vi "getStatus.vi"(8 "error in (no error)":errorcluster, 11 "SpinCore in":refnum<class "SpinCore.lvclass">) -> (0 "error out":errorcluster, 2 "status array":bool[](array[boolean]), 3 "SpinCore out":refnum<class "SpinCore.lvclass">)   [LabVIEW 2009, in "Hardware.lvlib" / "Channels.lvlib" / "SpinCore.lvclass"]
uses:
  SpinCore.lvclass
  SpinCore.lvclass/SpinCore.ctl
panel:
  # "pb_read_status(void) returns a 32 bit int:\nbit0 :stopped\nbit1: Reset\nbit2:Running\nbit3: Waiting\nBit4: Scanning (not this board)\nBit5-31 are reserved for future use.\n\nSee SpinAPI reference for details"
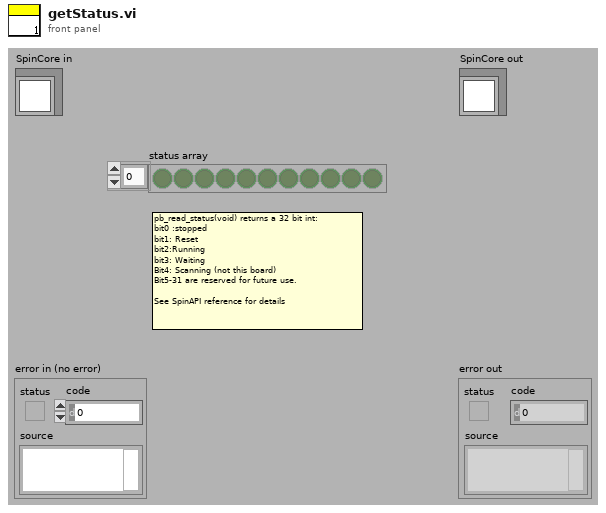
[diagram p1: front panel]
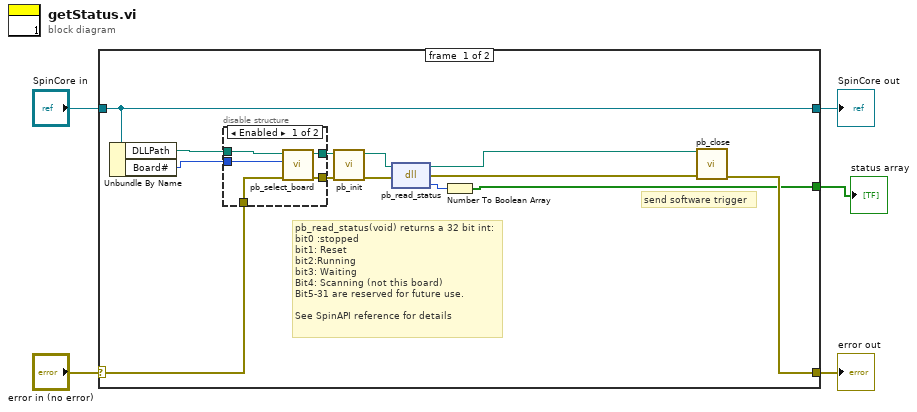
[diagram p0: block diagram]
diagram:
  n1 = case shown="No Error" "error in (no error)" {
    selector: "error in (no error)" -> [w15 w27]
    tunnel: [w7 w27] -> w4
    tunnel: [w18 w26] -> w2
    tunnel: "SpinCore in" -> [w18 w26]
    tunnel: [w6 _] -> w1
    frame #0 {
      # "pb_read_status(void) returns a 32 bit int:\nbit0 :stopped\nbit1: Reset\nbit2:Running\nbit3: Waiting\nBit4: Scanning (not this board)\nBit5-31 are reserved for future use.\n\nSee SpinAPI reference for details"
      # "send software trigger"
      n2 = Unbundle By Name(w18) -> ("DLLPath"=w17:path, "Board#"=w16:i32)
      n3 = disable-structure shown="Enabled" {
        disable-tunnel: w17 -> [w23 w25]
        disable-tunnel: w16 -> [w22 _]
        disable-tunnel: w15 -> [w21 w24]
        disable-tunnel: [w20 w24] -> w14
        disable-tunnel: [w19 w25] -> w13
        frame #0 {
          n4 = call <userlib>:"pb_select_board.vi"("error in (no error)"=w21, "board_num"=w22, "path in"=w23) -> ("error out"=w20:errorcluster, "path out"=w19:path)  [unwired: 7 in]
        }
        frame #1 {
        }
      }
      n5 = call <userlib>:"pb_init.vi"("error in (no error)"=w14, "path in"=w13) -> ("error out"=w12:errorcluster, "path out"=w11:path)  [unwired: 8 in]
      n6 = dll-call lib="C:/Program Files/National Instruments/LabVIEW 2009/spinapi.dll" fn="pb_read_status"(path in=w11, error in=w12) -> (path out=w9:path, error out=w8:errorcluster, "status"=w10:i32)  [unwired: 1 in]
      n7 = Number To Boolean Array(number=w10) -> (Boolean array=w6:bool[])
      n8 = call <userlib>:"pb_close.vi"("error in (no error)"=w8, "path in"=w9) -> ("error out"=w7:errorcluster)  [unwired: 8 in, 1 out]
    }
    frame #1 {
    }
  }
  "error out" <- w4
  "SpinCore out" <- w2
  "status array" <- w1
